vi "Custom Failure Message.vi"() -> ()   [LabVIEW 2017, in "Assertions.Tests.lvlib" / "Assert Refnum.lvlib"]
uses:
  Assert Refnum.lvlib
  src/Transparent Assertions/Assertions/Assertions.lvlib
panel:
  out "error out":errorcluster
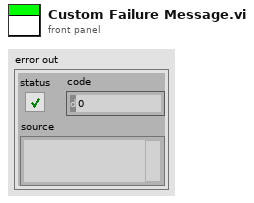
[diagram p1: front panel]
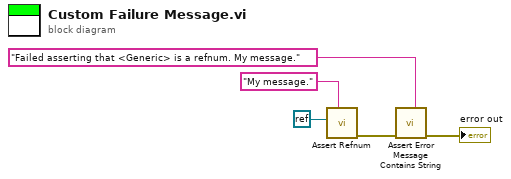
[diagram p0: block diagram]
diagram:
  n1 = call "Assert Refnum.vi"("Message (\"\")"="My message." ("Message (\"\")"), "Refnum"=refnum<k0> refnum) -> ("error out"=w5:errorcluster)  [unwired: 9 in]
  n2 = call "Assert Error Message Contains String.vi"("Expected"="Failed asserting that <Generic> is a refnum. My message.", "error in (no error)"=w5) -> ("error out"=→"error out":errorcluster)  [unwired: 9 in]
